vi "Motor_Init.vi"   [LabVIEW 2019]
uses:
  Globals/Drive_Globals.vi
  <vilib>/Rock Robotics/WPI/ThirdParty/Phoenix-LabVIEW/Motor Controller/Controls/CTRE_Phoenix_MotorControl_ControlMode.ctl
  <vilib>/Rock Robotics/WPI/ThirdParty/Phoenix-LabVIEW/Motor Controller/Controls/CTRE_Phoenix_MotorControl_FeedbackDevice.ctl
types:
  T1 = typedef "CTRE_Phoenix_MotorControl_FeedbackDevice.ctl" = i8
  T2 = typedef "CTRE_Phoenix_MotorControl_ControlMode.ctl" = u16
  T3 = typedef "WPI_MotorControlDeviceRef.ctl" = cluster{"DeviceStatus":errorcluster, "Type":T4, "PWM":cluster{"PWM Channel":T5, "DeadBand":T6}, "CAN":cluster{"Device Number":u8, "SetOutput VI Ref":variant, "GetOutput VI Ref":variant, "Enable VI Ref":variant, "Disable VI Ref":variant, "Data":variant}, "Invert":bool, "DIO PWM":cluster{"PWM \"Enable\" Channel":T5, "DIOChannel":T7, "PWM Rate":dbl}}
  T4 = typedef "WPI_MotorControlType.ctl" = enum16{"PWM", "CAN", "DIO PWM"}
  T5 = typedef "FPGA_DIOPWMChannel.ctl" = enum8{"PWM 0", "PWM 1", "PWM 2", "PWM 3", "PWM 4", "PWM 5", "PWM 6", "PWM 7", "PWM 8", "PWM 9", "PWM MXP 0", "PWM MXP 1", "PWM MXP 2", "PWM MXP 3", "PWM MXP 4", "PWM MXP 5", "PWM MXP 6", "PWM MXP 7", "PWM MXP 8", "PWM MXP 9", "Invalid"}
  T6 = typedef "WPI_PWMDeadband.ctl" = cluster{"Name":string, "maxPositivePwm":i32, "minPositivePwm":i32, "centerPwm":i32, "maxNegativePwm":i32, "minNegativePwm":i32, "angularRange":u16}
  T7 = typedef "FPGA_DIOChannel.ctl" = enum8{"DIO 0", "DIO 1", "DIO 2", "DIO 3", "DIO 4", "DIO 5", "DIO 6", "DIO 7", "DIO 8", "DIO 9", "DIO MXP 0", "DIO MXP 1", "DIO MXP 2", "DIO MXP 3", "DIO MXP 4", "DIO MXP 5", "DIO MXP 6", "DIO MXP 7", "DIO MXP 8", "DIO MXP 9", "DIO MXP 10", "DIO MXP 11", "DIO MXP 12", "DIO MXP 13", "DIO MXP 14", "DIO MXP 15", "SPI Port CS1", "SPI Port CS2", "SPI Port CS3", "SPI Port MISO", "SPI Port MOSI", "Invalid"}
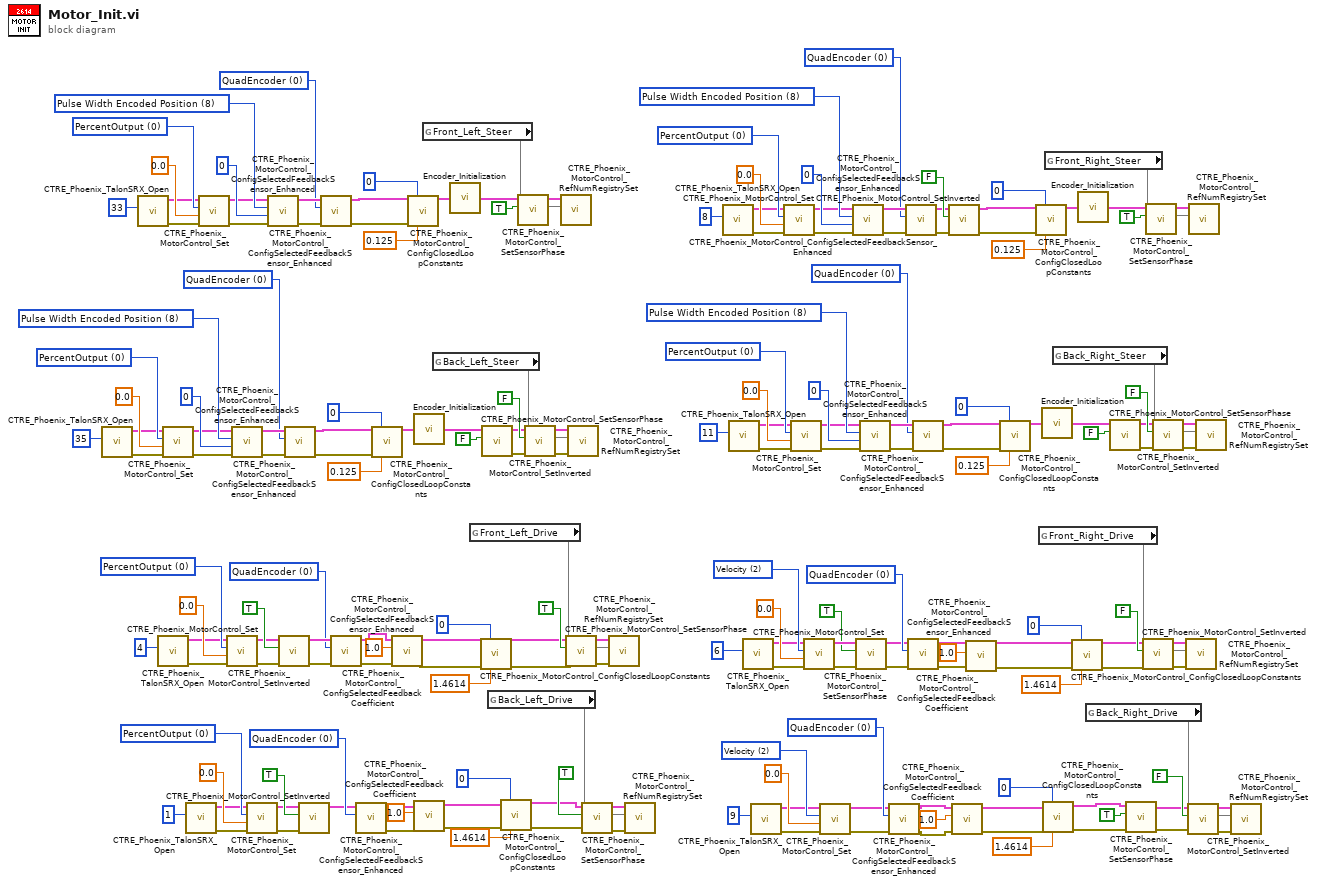
[diagram p0: block diagram]
diagram:
  w46 = T1 0 items=["None"=-1, "QuadEncoder"=0, "Analog"=2, "Tachometer"=4, "Pulse Width Encoded Position"=8, "Sensor Sum (S0 + S1)"=9, "Sensor Difference (D0 - D1)"=10, "Remote Source 0"=11, "Remote Source 1"=12, "Software Emulated"=15] ("Feedback Device")
  w54 = T1 0 items=["None"=-1, "QuadEncoder"=0, "Analog"=2, "Tachometer"=4, "Pulse Width Encoded Position"=8, "Sensor Sum (S0 + S1)"=9, "Sensor Difference (D0 - D1)"=10, "Remote Source 0"=11, "Remote Source 1"=12, "Software Emulated"=15] ("Feedback Device")
  w55 = T1 0 items=["None"=-1, "QuadEncoder"=0, "Analog"=2, "Tachometer"=4, "Pulse Width Encoded Position"=8, "Sensor Sum (S0 + S1)"=9, "Sensor Difference (D0 - D1)"=10, "Remote Source 0"=11, "Remote Source 1"=12, "Software Emulated"=15] ("Feedback Device")
  w57 = T1 0 items=["None"=-1, "QuadEncoder"=0, "Analog"=2, "Tachometer"=4, "Pulse Width Encoded Position"=8, "Sensor Sum (S0 + S1)"=9, "Sensor Difference (D0 - D1)"=10, "Remote Source 0"=11, "Remote Source 1"=12, "Software Emulated"=15] ("Feedback Device")
  w78 = T2 0 items=["PercentOutput"=0, "Position"=1, "Velocity"=2, "Current"=3, "Follower"=5, "MotionProfile"=6, "MotionMagic"=7, "MotionMagicArc"=8, "MotionProfileArc"=10, "Disabled"=15] ("Control Mode")
  w83 = T2 0 items=["PercentOutput"=0, "Position"=1, "Velocity"=2, "Current"=3, "Follower"=5, "MotionProfile"=6, "MotionMagic"=7, "MotionMagicArc"=8, "MotionProfileArc"=10, "Disabled"=15] ("Control Mode")
  w88 = T2 2 items=["PercentOutput"=0, "Position"=1, "Velocity"=2, "Current"=3, "Follower"=5, "MotionProfile"=6, "MotionMagic"=7, "MotionMagicArc"=8, "MotionProfileArc"=10, "Disabled"=15] ("Control Mode")
  w93 = T2 2 items=["PercentOutput"=0, "Position"=1, "Velocity"=2, "Current"=3, "Follower"=5, "MotionProfile"=6, "MotionMagic"=7, "MotionMagicArc"=8, "MotionProfileArc"=10, "Disabled"=15] ("Control Mode")
  w120 = T1 0 items=["None"=-1, "QuadEncoder"=0, "Analog"=2, "Tachometer"=4, "Pulse Width Encoded Position"=8, "Sensor Sum (S0 + S1)"=9, "Sensor Difference (D0 - D1)"=10, "Remote Source 0"=11, "Remote Source 1"=12, "Software Emulated"=15] ("Feedback Device")
  w124 = T1 0 items=["None"=-1, "QuadEncoder"=0, "Analog"=2, "Tachometer"=4, "Pulse Width Encoded Position"=8, "Sensor Sum (S0 + S1)"=9, "Sensor Difference (D0 - D1)"=10, "Remote Source 0"=11, "Remote Source 1"=12, "Software Emulated"=15] ("Feedback Device")
  w129 = T1 0 items=["None"=-1, "QuadEncoder"=0, "Analog"=2, "Tachometer"=4, "Pulse Width Encoded Position"=8, "Sensor Sum (S0 + S1)"=9, "Sensor Difference (D0 - D1)"=10, "Remote Source 0"=11, "Remote Source 1"=12, "Software Emulated"=15] ("Feedback Device")
  w135 = T1 0 items=["None"=-1, "QuadEncoder"=0, "Analog"=2, "Tachometer"=4, "Pulse Width Encoded Position"=8, "Sensor Sum (S0 + S1)"=9, "Sensor Difference (D0 - D1)"=10, "Remote Source 0"=11, "Remote Source 1"=12, "Software Emulated"=15] ("Feedback Device")
  w155 = T1 8 items=["None"=-1, "QuadEncoder"=0, "Analog"=2, "Tachometer"=4, "Pulse Width Encoded Position"=8, "Sensor Sum (S0 + S1)"=9, "Sensor Difference (D0 - D1)"=10, "Remote Source 0"=11, "Remote Source 1"=12, "Software Emulated"=15] ("Feedback Device")
  w150 = T2 0 items=["PercentOutput"=0, "Position"=1, "Velocity"=2, "Current"=3, "Follower"=5, "MotionProfile"=6, "MotionMagic"=7, "MotionMagicArc"=8, "MotionProfileArc"=10, "Disabled"=15] ("Control Mode")
  w166 = T1 8 items=["None"=-1, "QuadEncoder"=0, "Analog"=2, "Tachometer"=4, "Pulse Width Encoded Position"=8, "Sensor Sum (S0 + S1)"=9, "Sensor Difference (D0 - D1)"=10, "Remote Source 0"=11, "Remote Source 1"=12, "Software Emulated"=15] ("Feedback Device")
  w161 = T2 0 items=["PercentOutput"=0, "Position"=1, "Velocity"=2, "Current"=3, "Follower"=5, "MotionProfile"=6, "MotionMagic"=7, "MotionMagicArc"=8, "MotionProfileArc"=10, "Disabled"=15] ("Control Mode")
  w177 = T1 8 items=["None"=-1, "QuadEncoder"=0, "Analog"=2, "Tachometer"=4, "Pulse Width Encoded Position"=8, "Sensor Sum (S0 + S1)"=9, "Sensor Difference (D0 - D1)"=10, "Remote Source 0"=11, "Remote Source 1"=12, "Software Emulated"=15] ("Feedback Device")
  w172 = T2 0 items=["PercentOutput"=0, "Position"=1, "Velocity"=2, "Current"=3, "Follower"=5, "MotionProfile"=6, "MotionMagic"=7, "MotionMagicArc"=8, "MotionProfileArc"=10, "Disabled"=15] ("Control Mode")
  w188 = T1 8 items=["None"=-1, "QuadEncoder"=0, "Analog"=2, "Tachometer"=4, "Pulse Width Encoded Position"=8, "Sensor Sum (S0 + S1)"=9, "Sensor Difference (D0 - D1)"=10, "Remote Source 0"=11, "Remote Source 1"=12, "Software Emulated"=15] ("Feedback Device")
  w183 = T2 0 items=["PercentOutput"=0, "Position"=1, "Velocity"=2, "Current"=3, "Follower"=5, "MotionProfile"=6, "MotionMagic"=7, "MotionMagicArc"=8, "MotionProfileArc"=10, "Disabled"=15] ("Control Mode")
  n1 = call <vilib>:"CTRE_Phoenix_TalonSRX_Open.vi"("Device Number"=u8 35) -> ("error out"=w174:errorcluster, "CAN Talon SRX Ref"=w171:T3)  [unwired: 9 in]
  n2 = call <vilib>:"CTRE_Phoenix_TalonSRX_Open.vi"("Device Number"=u8 33) -> ("error out"=w185:errorcluster, "CAN Talon SRX Ref"=w182:T3)  [unwired: 9 in]
  n3 = call <vilib>:"CTRE_Phoenix_TalonSRX_Open.vi"("Device Number"=u8 4) -> ("error out"=w36:errorcluster, "CAN Talon SRX Ref"=w37:T3)  [unwired: 9 in]
  n4 = call <vilib>:"CTRE_Phoenix_MotorControl_Set.vi"("error in (no error)"=w174, "Output"=0.0, "Control Mode"=w172, "PhoenixMotorControlDevRef"=w171) -> ("error out"=w176:errorcluster, "PhoenixMotorControlDevRef"=w175:T3)  [unwired: 6 in]
  n5 = call <vilib>:"CTRE_Phoenix_TalonSRX_Open.vi"("Device Number"=u8 1) -> ("error out"=w80:errorcluster, "CAN Talon SRX Ref"=w77:T3)  [unwired: 9 in]
  n6 = call <vilib>:"CTRE_Phoenix_MotorControl_Set.vi"("error in (no error)"=w185, "Output"=0.0, "Control Mode"=w183, "PhoenixMotorControlDevRef"=w182) -> ("error out"=w187:errorcluster, "PhoenixMotorControlDevRef"=w186:T3)  [unwired: 6 in]
  n7 = call <vilib>:"CTRE_Phoenix_MotorControl_Set.vi"("error in (no error)"=w36, "Output"=0.0, "Control Mode"=w83, "PhoenixMotorControlDevRef"=w37) -> ("error out"=w73:errorcluster, "PhoenixMotorControlDevRef"=w74:T3)  [unwired: 6 in]
  n8 = call <vilib>:"CTRE_Phoenix_MotorControl_ConfigSelectedFeedbackSensor_Enhanced.vi"("error in (no error)"=w176, "pidLoopIdx"=0, "Feedback Device"=w177, "PhoenixMotorControlDevRef"=w175) -> ("error out"=w132:errorcluster, "PhoenixMotorControlDevRef"=w133:T3)  [unwired: 6 in]
  n9 = call <vilib>:"CTRE_Phoenix_MotorControl_Set.vi"("error in (no error)"=w80, "Output"=0.0, "Control Mode"=w78, "PhoenixMotorControlDevRef"=w77) -> ("error out"=w70:errorcluster, "PhoenixMotorControlDevRef"=w71:T3)  [unwired: 6 in]
  n10 = call <vilib>:"CTRE_Phoenix_MotorControl_ConfigSelectedFeedbackSensor_Enhanced.vi"("error in (no error)"=w187, "pidLoopIdx"=0, "Feedback Device"=w188, "PhoenixMotorControlDevRef"=w186) -> ("error out"=w138:errorcluster, "PhoenixMotorControlDevRef"=w139:T3)  [unwired: 6 in]
  n11 = call <vilib>:"CTRE_Phoenix_MotorControl_SetInverted.vi"("error in (no error)"=w73, "Invert?"=TRUE, "PhoenixMotorControlDevRef"=w74) -> ("error out"=w50:errorcluster, "PhoenixMotorControlDevRef"=w49:T3)  [unwired: 7 in]
  n12 = call <vilib>:"CTRE_Phoenix_MotorControl_ConfigSelectedFeedbackSensor_Enhanced.vi"("error in (no error)"=w132, "Feedback Device"=w129, "PhoenixMotorControlDevRef"=w133) -> ("error out"=w130:errorcluster, "PhoenixMotorControlDevRef"=w131:T3)  [unwired: 7 in]
  n13 = call <vilib>:"CTRE_Phoenix_MotorControl_SetInverted.vi"("error in (no error)"=w70, "Invert?"=TRUE, "PhoenixMotorControlDevRef"=w71) -> ("PhoenixMotorControlDevRef"=w56:T3)  [unwired: 7 in, 1 out]
  n14 = call <vilib>:"CTRE_Phoenix_MotorControl_ConfigSelectedFeedbackSensor_Enhanced.vi"("error in (no error)"=w138, "Feedback Device"=w135, "PhoenixMotorControlDevRef"=w139) -> ("error out"=w136:errorcluster, "PhoenixMotorControlDevRef"=w137:T3)  [unwired: 7 in]
  n15 = call <vilib>:"CTRE_Phoenix_MotorControl_ConfigSelectedFeedbackSensor_Enhanced.vi"("error in (no error)"=w50, "Feedback Device"=w46, "PhoenixMotorControlDevRef"=w49) -> ("error out"=w7:errorcluster, "PhoenixMotorControlDevRef"=w8:T3)  [unwired: 7 in]
  n16 = call <vilib>:"CTRE_Phoenix_MotorControl_ConfigSelectedFeedbackSensor_Enhanced.vi"("Feedback Device"=w57, "PhoenixMotorControlDevRef"=w56) -> ("error out"=w38:errorcluster, "PhoenixMotorControlDevRef"=w39:T3)  [unwired: 8 in]
  n17 = call <vilib>:"CTRE_Phoenix_MotorControl_ConfigClosedLoopConstants.vi"("PhoenixMotorControlDevRef"=w131, "slotIdx"=0, "error in (no error)"=w130, "F"=0.125) -> ("PhoenixMotorControlDevRef"=w116:T3)  [unwired: 10 in, 1 out]
  n18 = call <vilib>:"CTRE_Phoenix_MotorControl_ConfigSelectedFeedbackCoefficient.vi"("error in (no error)"=w7, "coefficient"=1.0, "PhoenixMotorControlDevRef"=w8) -> ("error out"=w3:errorcluster, "PhoenixMotorControlDevRef"=w4:T3)  [unwired: 7 in]
  n19 = call <vilib>:"CTRE_Phoenix_MotorControl_ConfigClosedLoopConstants.vi"("PhoenixMotorControlDevRef"=w137, "slotIdx"=0, "error in (no error)"=w136, "F"=0.125) -> ("PhoenixMotorControlDevRef"=w134:T3)  [unwired: 10 in, 1 out]
  n20 = call "Encoder_Initialization.vi"("Ref In"=w116) -> ("Ref Out"=w115:T3)
  n21 = call <vilib>:"CTRE_Phoenix_MotorControl_ConfigSelectedFeedbackCoefficient.vi"("error in (no error)"=w38, "coefficient"=1.0, "PhoenixMotorControlDevRef"=w39) -> ("error out"=w12:errorcluster, "PhoenixMotorControlDevRef"=w13:T3)  [unwired: 7 in]
  n22 = global read "Drive_Globals.vi" "Front_Left_Steer"() -> (w143)
  n23 = global read "Drive_Globals.vi" "Back_Left_Steer"() -> (w180)
  n24 = call "Encoder_Initialization.vi"("Ref In"=w134) -> ("Ref Out"=w112:T3)
  n25 = global read "Drive_Globals.vi" "Front_Left_Drive"() -> (w85)
  n26 = call <vilib>:"CTRE_Phoenix_MotorControl_ConfigClosedLoopConstants.vi"("PhoenixMotorControlDevRef"=w4, "slotIdx"=0, "error in (no error)"=w3, "F"=1.4614) -> ("PhoenixMotorControlDevRef"=w1:T3, "error out"=w2:errorcluster)  [unwired: 10 in]
  n27 = call <vilib>:"CTRE_Phoenix_MotorControl_SetSensorPhase.vi"("PhaseSensor"=FALSE, "PhoenixMotorControlDevRef"=w115) -> ("error out"=w98:errorcluster, "PhoenixMotorControlDevRef"=w99:T3)  [unwired: 8 in]
  n28 = global read "Drive_Globals.vi" "Back_Left_Drive"() -> (w81)
  n29 = call <vilib>:"CTRE_Phoenix_MotorControl_ConfigClosedLoopConstants.vi"("PhoenixMotorControlDevRef"=w13, "slotIdx"=0, "error in (no error)"=w12, "F"=1.4614) -> ("PhoenixMotorControlDevRef"=w10:T3, "error out"=w11:errorcluster)  [unwired: 10 in]
  n30 = call <vilib>:"CTRE_Phoenix_MotorControl_SetSensorPhase.vi"("PhaseSensor"=TRUE, "PhoenixMotorControlDevRef"=w112) -> ("PhoenixMotorControlDevRef"=w111:T3)  [unwired: 8 in, 1 out]
  n31 = call <vilib>:"CTRE_Phoenix_MotorControl_SetInverted.vi"("error in (no error)"=w98, "Invert?"=FALSE, "PhoenixMotorControlDevRef"=w99) -> ("error out"=w97:errorcluster, "PhoenixMotorControlDevRef"=w96:T3)  [unwired: 7 in]
  n32 = call <vilib>:"CTRE_Phoenix_MotorControl_RefNumRegistrySet.vi"("refnum name"=w143, "PhoenixMotorControlDevRef"=w111) -> ()  [unwired: 8 in, 2 out]
  n33 = call <vilib>:"CTRE_Phoenix_MotorControl_SetSensorPhase.vi"("error in (no error)"=w2, "PhaseSensor"=TRUE, "PhoenixMotorControlDevRef"=w1) -> ("error out"=w47:errorcluster, "PhoenixMotorControlDevRef"=w48:T3)  [unwired: 7 in]
  n34 = call <vilib>:"CTRE_Phoenix_MotorControl_RefNumRegistrySet.vi"("error in (no error)"=w97, "refnum name"=w180, "PhoenixMotorControlDevRef"=w96) -> ()  [unwired: 7 in, 2 out]
  n35 = call <vilib>:"CTRE_Phoenix_MotorControl_SetSensorPhase.vi"("error in (no error)"=w11, "PhaseSensor"=TRUE, "PhoenixMotorControlDevRef"=w10) -> ("error out"=w62:errorcluster, "PhoenixMotorControlDevRef"=w63:T3)  [unwired: 7 in]
  n36 = call <vilib>:"CTRE_Phoenix_MotorControl_RefNumRegistrySet.vi"("error in (no error)"=w47, "refnum name"=w85, "PhoenixMotorControlDevRef"=w48) -> ()  [unwired: 7 in, 2 out]
  n37 = call <vilib>:"CTRE_Phoenix_MotorControl_RefNumRegistrySet.vi"("error in (no error)"=w62, "refnum name"=w81, "PhoenixMotorControlDevRef"=w63) -> ()  [unwired: 7 in, 2 out]
  n38 = call <vilib>:"CTRE_Phoenix_TalonSRX_Open.vi"("Device Number"=u8 8) -> ("error out"=w163:errorcluster, "CAN Talon SRX Ref"=w160:T3)  [unwired: 9 in]
  n39 = call <vilib>:"CTRE_Phoenix_TalonSRX_Open.vi"("Device Number"=u8 11) -> ("error out"=w152:errorcluster, "CAN Talon SRX Ref"=w149:T3)  [unwired: 9 in]
  n40 = call <vilib>:"CTRE_Phoenix_TalonSRX_Open.vi"("Device Number"=u8 6) -> ("error out"=w41:errorcluster, "CAN Talon SRX Ref"=w42:T3)  [unwired: 9 in]
  n41 = call <vilib>:"CTRE_Phoenix_TalonSRX_Open.vi"("Device Number"=u8 9) -> ("error out"=w90:errorcluster, "CAN Talon SRX Ref"=w87:T3)  [unwired: 9 in]
  n42 = call <vilib>:"CTRE_Phoenix_MotorControl_Set.vi"("error in (no error)"=w163, "Output"=0.0, "Control Mode"=w161, "PhoenixMotorControlDevRef"=w160) -> ("error out"=w165:errorcluster, "PhoenixMotorControlDevRef"=w164:T3)  [unwired: 6 in]
  n43 = call <vilib>:"CTRE_Phoenix_MotorControl_Set.vi"("error in (no error)"=w152, "Output"=0.0, "Control Mode"=w150, "PhoenixMotorControlDevRef"=w149) -> ("error out"=w154:errorcluster, "PhoenixMotorControlDevRef"=w153:T3)  [unwired: 6 in]
  n44 = call <vilib>:"CTRE_Phoenix_MotorControl_Set.vi"("error in (no error)"=w41, "Output"=0.0, "Control Mode"=w93, "PhoenixMotorControlDevRef"=w42) -> ("error out"=w60:errorcluster, "PhoenixMotorControlDevRef"=w59:T3)  [unwired: 6 in]
  n45 = call <vilib>:"CTRE_Phoenix_MotorControl_Set.vi"("error in (no error)"=w90, "Output"=0.0, "Control Mode"=w88, "PhoenixMotorControlDevRef"=w87) -> ("error out"=w24:errorcluster, "PhoenixMotorControlDevRef"=w25:T3)  [unwired: 6 in]
  n46 = call <vilib>:"CTRE_Phoenix_MotorControl_ConfigSelectedFeedbackSensor_Enhanced.vi"("error in (no error)"=w165, "pidLoopIdx"=0, "Feedback Device"=w166, "PhoenixMotorControlDevRef"=w164) -> ("error out"=w121:errorcluster, "PhoenixMotorControlDevRef"=w122:T3)  [unwired: 6 in]
  n47 = call <vilib>:"CTRE_Phoenix_MotorControl_SetSensorPhase.vi"("error in (no error)"=w60, "PhaseSensor"=TRUE, "PhoenixMotorControlDevRef"=w59) -> ("error out"=w52:errorcluster, "PhoenixMotorControlDevRef"=w53:T3)  [unwired: 7 in]
  n48 = call <vilib>:"CTRE_Phoenix_MotorControl_ConfigSelectedFeedbackSensor_Enhanced.vi"("error in (no error)"=w154, "pidLoopIdx"=0, "Feedback Device"=w155, "PhoenixMotorControlDevRef"=w153) -> ("error out"=w127:errorcluster, "PhoenixMotorControlDevRef"=w128:T3)  [unwired: 6 in]
  n49 = call <vilib>:"CTRE_Phoenix_MotorControl_ConfigSelectedFeedbackSensor_Enhanced.vi"("error in (no error)"=w24, "Feedback Device"=w55, "PhoenixMotorControlDevRef"=w25) -> ("error out"=w22:errorcluster, "PhoenixMotorControlDevRef"=w23:T3)  [unwired: 7 in]
  n50 = call <vilib>:"CTRE_Phoenix_MotorControl_ConfigSelectedFeedbackSensor_Enhanced.vi"("error in (no error)"=w121, "Feedback Device"=w120, "PhoenixMotorControlDevRef"=w122) -> ("error out"=w117:errorcluster, "PhoenixMotorControlDevRef"=w118:T3)  [unwired: 7 in]
  n51 = call <vilib>:"CTRE_Phoenix_MotorControl_ConfigSelectedFeedbackSensor_Enhanced.vi"("error in (no error)"=w52, "Feedback Device"=w54, "PhoenixMotorControlDevRef"=w53) -> ("error out"=w33:errorcluster, "PhoenixMotorControlDevRef"=w34:T3)  [unwired: 7 in]
  n52 = call <vilib>:"CTRE_Phoenix_MotorControl_ConfigSelectedFeedbackSensor_Enhanced.vi"("error in (no error)"=w127, "Feedback Device"=w124, "PhoenixMotorControlDevRef"=w128) -> ("error out"=w126:errorcluster, "PhoenixMotorControlDevRef"=w125:T3)  [unwired: 7 in]
  n53 = call <vilib>:"CTRE_Phoenix_MotorControl_SetInverted.vi"("error in (no error)"=w117, "Invert?"=FALSE, "PhoenixMotorControlDevRef"=w118) -> ("error out"=w141:errorcluster, "PhoenixMotorControlDevRef"=w140:T3)  [unwired: 7 in]
  n54 = call <vilib>:"CTRE_Phoenix_MotorControl_ConfigSelectedFeedbackCoefficient.vi"("error in (no error)"=w22, "coefficient"=1.0, "PhoenixMotorControlDevRef"=w23) -> ("error out"=w18:errorcluster, "PhoenixMotorControlDevRef"=w19:T3)  [unwired: 7 in]
  n55 = call <vilib>:"CTRE_Phoenix_MotorControl_ConfigSelectedFeedbackCoefficient.vi"("error in (no error)"=w33, "coefficient"=1.0, "PhoenixMotorControlDevRef"=w34) -> ("error out"=w29:errorcluster, "PhoenixMotorControlDevRef"=w30:T3)  [unwired: 7 in]
  n56 = call <vilib>:"CTRE_Phoenix_MotorControl_ConfigClosedLoopConstants.vi"("PhoenixMotorControlDevRef"=w125, "slotIdx"=0, "error in (no error)"=w126, "F"=0.125) -> ("PhoenixMotorControlDevRef"=w123:T3)  [unwired: 10 in, 1 out]
  n57 = call <vilib>:"CTRE_Phoenix_MotorControl_ConfigClosedLoopConstants.vi"("PhoenixMotorControlDevRef"=w140, "slotIdx"=0, "error in (no error)"=w141, "F"=0.125) -> ("PhoenixMotorControlDevRef"=w119:T3)  [unwired: 10 in, 1 out]
  n58 = global read "Drive_Globals.vi" "Front_Right_Drive"() -> (w95)
  n59 = call "Encoder_Initialization.vi"("Ref In"=w123) -> ("Ref Out"=w109:T3)
  n60 = call <vilib>:"CTRE_Phoenix_MotorControl_ConfigClosedLoopConstants.vi"("PhoenixMotorControlDevRef"=w19, "slotIdx"=0, "error in (no error)"=w18, "F"=1.4614) -> ("PhoenixMotorControlDevRef"=w16:T3, "error out"=w17:errorcluster)  [unwired: 10 in]
  n61 = global read "Drive_Globals.vi" "Front_Right_Steer"() -> (w169)
  n62 = global read "Drive_Globals.vi" "Back_Right_Steer"() -> (w158)
  n63 = call <vilib>:"CTRE_Phoenix_MotorControl_ConfigClosedLoopConstants.vi"("PhoenixMotorControlDevRef"=w30, "slotIdx"=0, "error in (no error)"=w29, "F"=1.4614) -> ("PhoenixMotorControlDevRef"=w28:T3, "error out"=w27:errorcluster)  [unwired: 10 in]
  n64 = call "Encoder_Initialization.vi"("Ref In"=w119) -> ("Ref Out"=w108:T3)
  n65 = global read "Drive_Globals.vi" "Back_Right_Drive"() -> (w91)
  n66 = call <vilib>:"CTRE_Phoenix_MotorControl_SetSensorPhase.vi"("PhaseSensor"=FALSE, "PhoenixMotorControlDevRef"=w109) -> ("error out"=w103:errorcluster, "PhoenixMotorControlDevRef"=w104:T3)  [unwired: 8 in]
  n67 = call <vilib>:"CTRE_Phoenix_MotorControl_SetSensorPhase.vi"("error in (no error)"=w17, "PhaseSensor"=TRUE, "PhoenixMotorControlDevRef"=w16) -> ("error out"=w44:errorcluster, "PhoenixMotorControlDevRef"=w43:T3)  [unwired: 7 in]
  n68 = call <vilib>:"CTRE_Phoenix_MotorControl_SetInverted.vi"("error in (no error)"=w27, "Invert?"=FALSE, "PhoenixMotorControlDevRef"=w28) -> ("error out"=w66:errorcluster, "PhoenixMotorControlDevRef"=w65:T3)  [unwired: 7 in]
  n69 = call <vilib>:"CTRE_Phoenix_MotorControl_SetSensorPhase.vi"("PhaseSensor"=TRUE, "PhoenixMotorControlDevRef"=w108) -> ("PhoenixMotorControlDevRef"=w107:T3)  [unwired: 8 in, 1 out]
  n70 = call <vilib>:"CTRE_Phoenix_MotorControl_SetInverted.vi"("error in (no error)"=w103, "Invert?"=FALSE, "PhoenixMotorControlDevRef"=w104) -> ("error out"=w102:errorcluster, "PhoenixMotorControlDevRef"=w101:T3)  [unwired: 7 in]
  n71 = call <vilib>:"CTRE_Phoenix_MotorControl_RefNumRegistrySet.vi"("error in (no error)"=w66, "refnum name"=w95, "PhoenixMotorControlDevRef"=w65) -> ()  [unwired: 7 in, 2 out]
  n72 = call <vilib>:"CTRE_Phoenix_MotorControl_SetInverted.vi"("error in (no error)"=w44, "Invert?"=FALSE, "PhoenixMotorControlDevRef"=w43) -> ("error out"=w68:errorcluster, "PhoenixMotorControlDevRef"=w67:T3)  [unwired: 7 in]
  n73 = call <vilib>:"CTRE_Phoenix_MotorControl_RefNumRegistrySet.vi"("refnum name"=w169, "PhoenixMotorControlDevRef"=w107) -> ()  [unwired: 8 in, 2 out]
  n74 = call <vilib>:"CTRE_Phoenix_MotorControl_RefNumRegistrySet.vi"("error in (no error)"=w102, "refnum name"=w158, "PhoenixMotorControlDevRef"=w101) -> ()  [unwired: 7 in, 2 out]
  n75 = call <vilib>:"CTRE_Phoenix_MotorControl_RefNumRegistrySet.vi"("error in (no error)"=w68, "refnum name"=w91, "PhoenixMotorControlDevRef"=w67) -> ()  [unwired: 7 in, 2 out]
